vi "Child Nodes Content.vi"(7 "Context":refnum<class "Context.lvclass">, 8 "Error In":errorcluster, 11 "Children":refnum<class "Abstract.lvclass">[](array[class])) -> (0 "Error Out":errorcluster, 3 "Content":string)   [LabVIEW 2018, in "Toolkit.lvlib" / "Nodes.lvlib" / "Section.lvclass"]
uses:
  Section.lvclass
  Abstract/Abstract.lvclass
  Data/Context/Context.lvclass
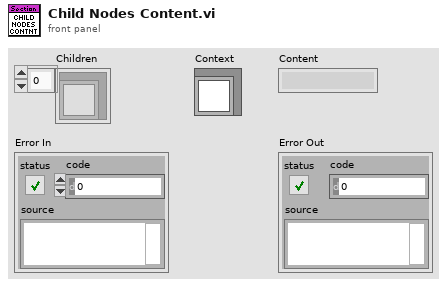
[diagram p1: front panel]
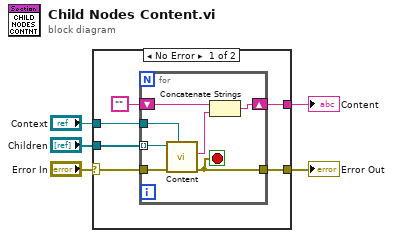
[diagram p0: block diagram]
diagram:
  n1 = case shown="No Error" "Error In" {
    selector: "Error In" -> [w6 w19]
    tunnel: "Children" -> [w11 _]
    tunnel: "Context" -> [w10 _]
    tunnel: [w9 w19] -> w3
    tunnel: [w7 _] -> w2
    frame No Error {
      n2 = for {
        tunnel: w6 -> [w18]
        tunnel: w11 -> [w17] mode=indexing
        tunnel: w10 -> [w16]
        tunnel: [w12] -> w9
        shift-right: [w13] -> w7
        shift-left: "" -> [w15]
        stop <- w12 stop-if-true
        n3 = call-dynamic "Content.vi"("Context"=w16, "Error In"=w18, "Abstract In"=w17) -> ("Error Out"=w12:errorcluster, "Content"=w14:string)  [unwired: 6 in, 1 out]
        n4 = Concatenate Strings(w15, w14) -> (w13:string)
      }
    }
    frame Error {
    }
  }
  "Error Out" <- w3
  "Content" <- w2
